vi "SubVIDemo.vi"() -> ()   [LabVIEW 2019]
panel:
  out "Number of Cents":dbl format="%#.2g"
  out "Dollar Value String":string
  out "?":dbl(knob) scale=0.0..10.0
  in  "Knob":dbl(knob) scale=0.0..1000.0
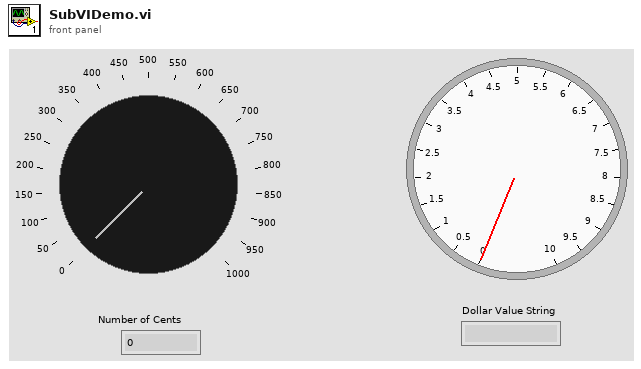
[diagram p1: front panel]
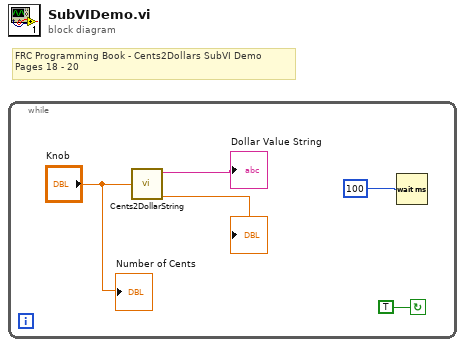
[diagram p0: block diagram]
diagram:
  # "FRC Programming Book - Cents2Dollars SubVI Demo\nPages 18 - 20"
  n1 = while {
    stop <- TRUE continue-if-true
    n2 = call "Cents2DollarString.vi"("Cents In"="Knob") -> ("Dollar Numeric Out"=→"?":dbl, "Dollar String Out"=→"Dollar Value String":string)  [unwired: 9 in]
    n3 = Wait (ms)(milliseconds to wait=100) -> ()  [unwired: 1 out]
    "Number of Cents" <- "Knob"
  }
